vi "CameraCtrlDEBUG.vi"(6 "Large cam coords":T1, 8 "error constant":errorcluster, 11 "Enum":enum16{"Start", "Stop", "Acquire", "Update"}(ring)) -> (0 "error constant 2":errorcluster, 3 "Large Camera":dbl[][](graph))   [LabVIEW 2019]
uses:
  CameraCoordsControl.ctl
panel:
  out "Camera connected":bool=TRUE
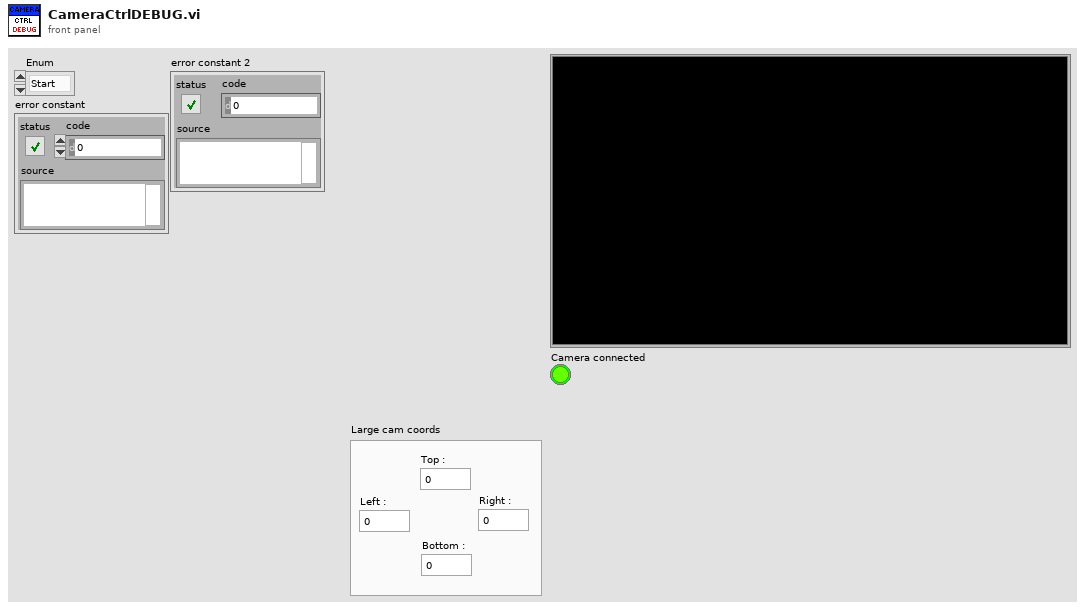
[diagram p1: front panel]
types:
  T1 = typedef "CameraCoordsControl.ctl" = cluster{"Top :":dbl, "Bottom :":dbl, "Left :":dbl, "Right :":dbl}
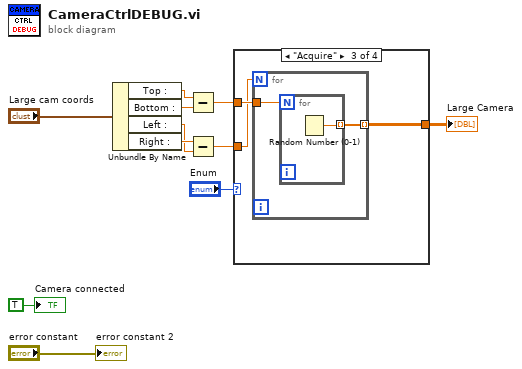
[diagram p0: block diagram]
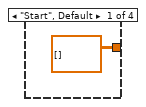
[diagram p2: hidden frame]
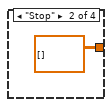
[diagram p3: hidden frame]
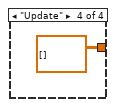
[diagram p4: hidden frame]
diagram:
  n1 = Unbundle By Name("Large cam coords") -> ("Top :"=w6:dbl, "Bottom :"=w5:dbl, "Left :"=w3:dbl, "Right :"=w4:dbl)
  n2 = Subtract(x=w6, y=w5) -> (x-y=w1:dbl)
  n3 = Subtract(x=w4, y=w3) -> (x-y=w2:dbl)
  n4 = case shown="\"Acquire\"" "Enum" {
    tunnel: [dbl[][] [] dbl[][] [] w16 dbl[][] []] -> w10
    tunnel: w2 -> [_ _ w14 _]
    tunnel: w1 -> [_ _ w15 _]
    frame "Start", Default {
    }
    frame "Stop" {
    }
    frame "Acquire" {
      n5 = for {
        N: w14 -> [_]
        tunnel: [w18] -> w16 mode=indexing
        tunnel: w15 -> [w17]
        n6 = for {
          N: w17 -> [_]
          tunnel: [w19] -> w18 mode=indexing
          n7 = Random Number (0-1)() -> (number: 0 to 1=w19:dbl)
        }
      }
    }
    frame "Update" {
    }
  }
  "Large Camera" <- w10
  "Camera connected" <- TRUE ("Camera connected")
  "error constant 2" <- "error constant"
